vi "Create All Message Queues.vi"(8 "error in (no error)":errorcluster) -> (0 "error out":errorcluster, 3 "Message Queues out":T1)   [LabVIEW 2020, in "Message Queue.lvlib"]
doc: "This VI creates and initializes all the message queues for your application. If your application requires more than one message queue, right-click the \"Message Queues\" constant above and select Open Type Def. Add the new Message Queue(s) to the type definition, then initialize them in this VI."
uses:
  Message Queue.lvlib
  All Message Queues.ctl
  Message Cluster.ctl
  Enqueue Message (Single).vi
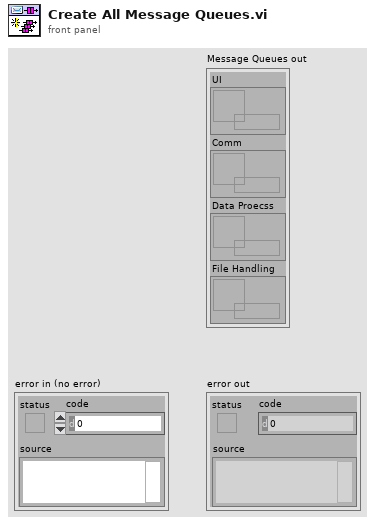
[diagram p1: front panel]
types:
  T1 = typedef "Message Queue.lvlib/All Message Queues.ctl" = cluster{"UI":refnum<queue>, "Comm":refnum<queue>, "Data Proecss":refnum<queue>, "File Handling":refnum<queue>}
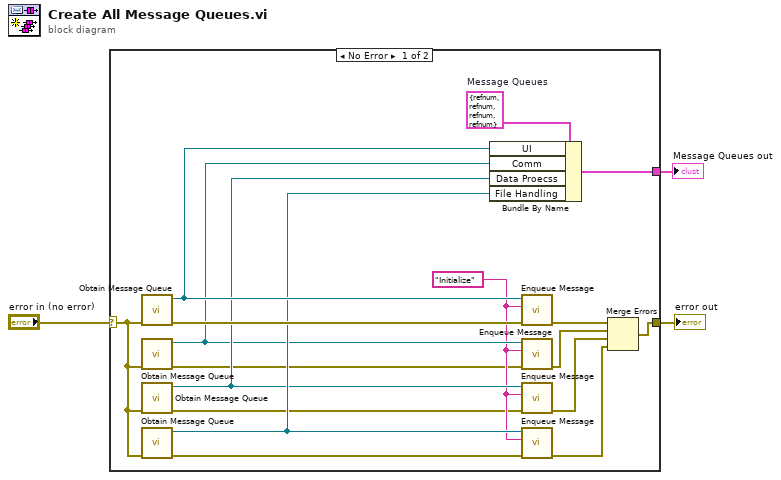
[diagram p0: block diagram]
diagram:
  n1 = case shown="No Error" "error in (no error)" {
    selector: "error in (no error)" -> [w11 w21]
    tunnel: [w7 w21] -> w3
    tunnel: [w18 _] -> w2
    frame No Error {
      w12 = "Initialize" ("Message")
      w19 = T1 {"UI"=refnum, "Comm"=refnum, "Data Proecss"=refnum, "File Handling"=refnum}  # Message Queues
      n2 = call "Obtain Message Queue.vi"("error in (no error)"=w11) -> ("error out"=w17:errorcluster, "Message Queue"=w16:refnum<queue>)  [unwired: 9 in]
      n3 = call "Obtain Message Queue.vi"("error in (no error)"=w11) -> ("error out"=w9:errorcluster, "Message Queue"=w13:refnum<queue>)  [unwired: 9 in]
      n4 = call "Obtain Message Queue.vi"("error in (no error)"=w11) -> ("error out"=w8:errorcluster, "Message Queue"=w14:refnum<queue>)  [unwired: 9 in]
      n5 = call "Obtain Message Queue.vi"("error in (no error)"=w11) -> ("error out"=w10:errorcluster, "Message Queue"=w15:refnum<queue>)  [unwired: 9 in]
      n6 = Bundle By Name(cluster=w19, "UI"=w16, "Comm"=w13, "Data Proecss"=w14, "File Handling"=w15) -> (w18:T1)
      n7 = call-poly "Enqueue Message.vi"("error in (no error)"=w17, "Message"=w12, "Message Queue"=w16) -> ("error out"=w20:errorcluster)  [unwired: 7 in, 1 out]
      n8 = call-poly "Enqueue Message.vi"("error in (no error)"=w9, "Message"=w12, "Message Queue"=w13) -> ("error out"=w6:errorcluster)  [unwired: 7 in, 1 out]
      n9 = call-poly "Enqueue Message.vi"("error in (no error)"=w8, "Message"=w12, "Message Queue"=w14) -> ("error out"=w5:errorcluster)  [unwired: 7 in, 1 out]
      n10 = call-poly "Enqueue Message.vi"("error in (no error)"=w10, "Message"=w12, "Message Queue"=w15) -> ("error out"=w4:errorcluster)  [unwired: 7 in, 1 out]
      n11 = Merge Errors(w20, w6, w5, w4) -> (w7:errorcluster)
    }
    frame Error {
    }
  }
  "Message Queues out" <- w2
  "error out" <- w3
